vi "rename libs.vi"(8 "error in (no error)":errorcluster, 10 "User Project":refnum<vi>, 11 "CD name":string) -> (0 "error out":errorcluster)   [LabVIEW 2014, in "CD model script.lvlib"]
uses:
  CD model script.lvlib
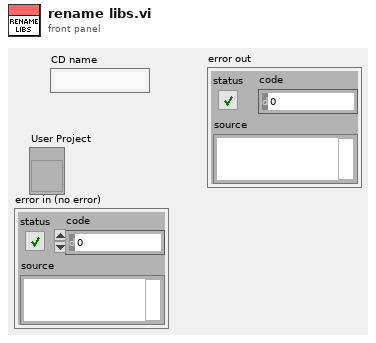
[diagram p1: front panel]
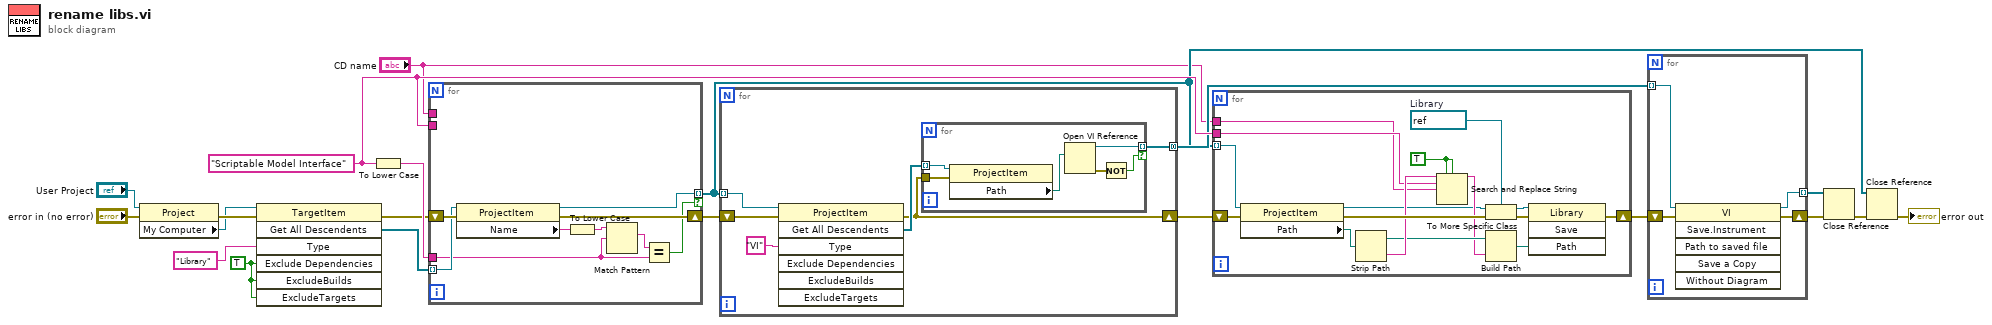
[diagram p0: block diagram]
diagram:
  w14 = TRUE ("ExcludeDependencies")
  w10 = "Scriptable Model Interface" ("Type")
  n1 = property class="Project"(reference="User Project", error in="error in (no error)") -> (error out=w17:errorcluster, "My Computer"=w15:refnum<vi>)  [unwired: 1 out]
  n2 = invoke class="TargetItem" method="Get All Descendents"(reference=w15, error in=w17, "Type"="Library", "Exclude Dependencies"=w14, "ExcludeBuilds"=w14, "ExcludeTargets"=w14) -> (error out=w18:errorcluster, "All Descendents"=w19:refnum<vi>[])  [unwired: 1 in, 5 out]
  n3 = To Lower Case(string=w10) -> (all lower case string=w20:string)
  n4 = for {
    shift-right: [w23] -> w12
    shift-left: w18 -> [w29]
    tunnel: w19 -> [w28] mode=indexing
    tunnel: w20 -> [w24]
    tunnel: w10 -> [_]
    tunnel: "CD name" -> [_]
    tunnel: [w22] -> w5 mode=indexing if=w21
    n5 = property class="ProjectItem"(reference=w28, error in=w29) -> (reference out=w22:refnum<vi>, error out=w23:errorcluster, "Name"=w27:string)
    n6 = To Lower Case(string=w27) -> (all lower case string=w26:string)
    n7 = Match Pattern(string=w26, regular expression=w24) -> (match substring=w25:string)  [unwired: 1 in, 3 out]
    n8 = Equal?(x=w25, y=w24) -> (x = y?=w21:bool)
  }
  n9 = for {
    shift-right: [w32] -> w11
    shift-left: w12 -> [w35]
    tunnel: w5 -> [w34] mode=indexing
    tunnel: [w31] -> w9 mode=concatenating
    n10 = invoke class="ProjectItem" method="Get All Descendents"(reference=w34, error in=w35, "Type"="VI") -> (error out=w32:errorcluster, "All Descendents"=w33:refnum<vi>[])  [unwired: 4 in, 5 out]
    n11 = for {
      tunnel: w33 -> [w41] mode=indexing
      tunnel: w32 -> [w40]
      tunnel: [w38] -> w31 mode=indexing if=w36
      n12 = property class="ProjectItem"(reference=w41, error in=w40) -> ("Path"=w39:path)  [unwired: 2 out]
      n13 = Open VI Reference(vi path=w39) -> (vi reference=w38:refnum<vi>, error out=w37:errorcluster)  [unwired: 5 in]
      n14 = Not(x=w37) -> (.not. x?=w36:bool)
    }
  }
  n15 = for {
    shift-right: [w43] -> w4
    shift-left: w11 -> [w57]
    tunnel: w5 -> [w46] mode=indexing
    tunnel: w10 -> [w48]
    tunnel: "CD name" -> [w47]
    w49 = TRUE ("replace all? (F)")
    w50 = refnum<vi> refnum  # Library
    n16 = property class="ProjectItem"(reference=w46, error in=w57) -> (reference out=w51:refnum<vi>, error out=w56:errorcluster, "Path"=w55:path)
    n17 = Strip Path(path=w55) -> (stripped path=w53:path, name=w54:string)
    n18 = Search and Replace String(replace all?=w49, case sensitive?=w49, input string=w54, search string=w48, replace string=w47) -> (result string=w52:string)  [unwired: 3 in, 3 out]
    n19 = To More Specific Class(target class=w50, reference=w51, error in=w56) -> (specific class reference=w44:refnum<vi>, error out=w45:errorcluster)
    n20 = Build Path(base path=w53, name or relative path=w52) -> (appended path=w42:path)
    n21 = invoke class="Library" method="Save"(reference=w44, error in=w45, "Path"=w42) -> (error out=w43:errorcluster)  [unwired: 1 in, 3 out]
  }
  n22 = for {
    tunnel: w9 -> [w60] mode=indexing
    tunnel: [w61] -> w6 mode=indexing
    shift-right: [w58] -> w3
    shift-left: w4 -> [w59]
    n23 = invoke class="VI" method="Save.Instrument"(reference=w60, error in=w59) -> (reference out=w61:refnum<vi>, error out=w58:errorcluster)  [unwired: 4 in, 4 out]
  }
  n24 = Close Reference(reference=w6, error in (no error)=w3) -> (error out=w8:errorcluster)
  n25 = Close Reference(reference=w5, error in (no error)=w8) -> (error out=→"error out":errorcluster)
